vi "索引数据.vi"(6 "引用簇":T1, 7 "簇输入":cluster{"数据":T3[], "显示数据":i32[]}, 8 "错误输入（无错误）":errorcluster) -> (0 "错误输出":errorcluster, 1 "突变电压":i32, 2 "测试类型":T2, 4 "数据":dbl[][](array[numeric]), 5 "簇输出":cluster{"数据":T3[], "显示数据":i32[]})   [LabVIEW 2021]
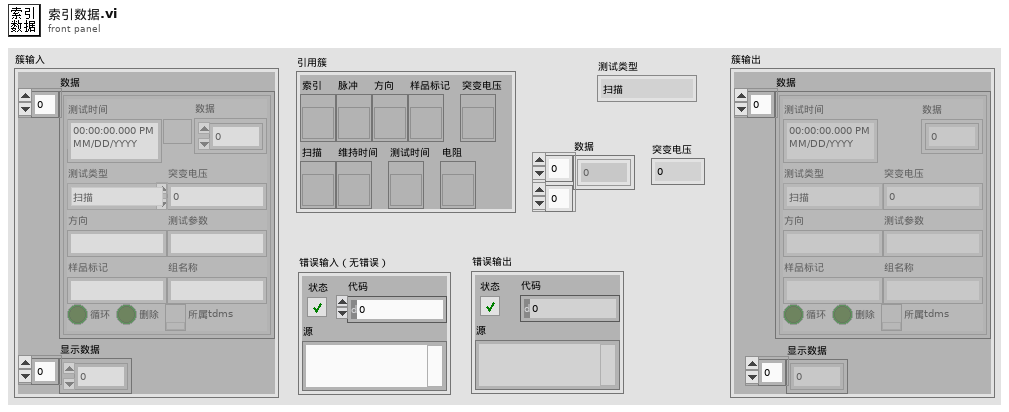
[diagram p1: front panel]
types:
  T1 = cluster{"索引":refnum<vi>, "扫描":refnum<vi>, "脉冲":refnum<vi>, "维持时间":refnum<vi>, "方向":refnum<vi>, "测试时间":refnum<vi>, "样品标记":refnum<vi>, "电阻":refnum<vi>, "突变电压":refnum<vi>}
  T2 = typedef "测试类型.ctl" = enum16{"扫描", "脉冲", "维持时间"}
  T3 = typedef "测试数据类型.ctl" = cluster{"测试时间":timestamp, "测试类型":T2, "方向":string, "样品标记":string, "测试参数":string, "循环":bool, "删除":bool, "组名称":string, "所属tdms":refnum<k34>, "突变电压":i32, "数据":dbl[][]}
  T4 = typedef "扫描参数.ctl" = cluster{"测试参数":cluster{"正向电压(V)":dbl, "正向极限电流(mA)":dbl, "反向电压(V)":dbl, "反向极限电流(mA)":dbl}, "时序参数":cluster{"正改变量(V)":dbl, "反改变量(V)":dbl, "维持时间(ms)":dbl, "nplc":dbl, "时序优先":bool}}
  T5 = typedef "脉冲参数.ctl" = cluster{"测试参数":cluster{"正向电压(V)":dbl, "正向极限电流(mA)":dbl, "反向电压(V)":dbl, "反向极限电流(mA)":dbl, "读取电压(V)":dbl}, "时序参数":cluster{"脉冲宽度(ms)":dbl, "脉冲间隔(ms)":dbl, "读取次数":u32}}
  T6 = typedef "维持时间.ctl" = cluster{"测试参数":cluster{"读取电压(V)":dbl, "极限电流(mA)":dbl}, "时序参数":cluster{"测试时间(s)":dbl, "读取间隔(ms)":dbl, "nplc":dbl, "时序优先":bool}}
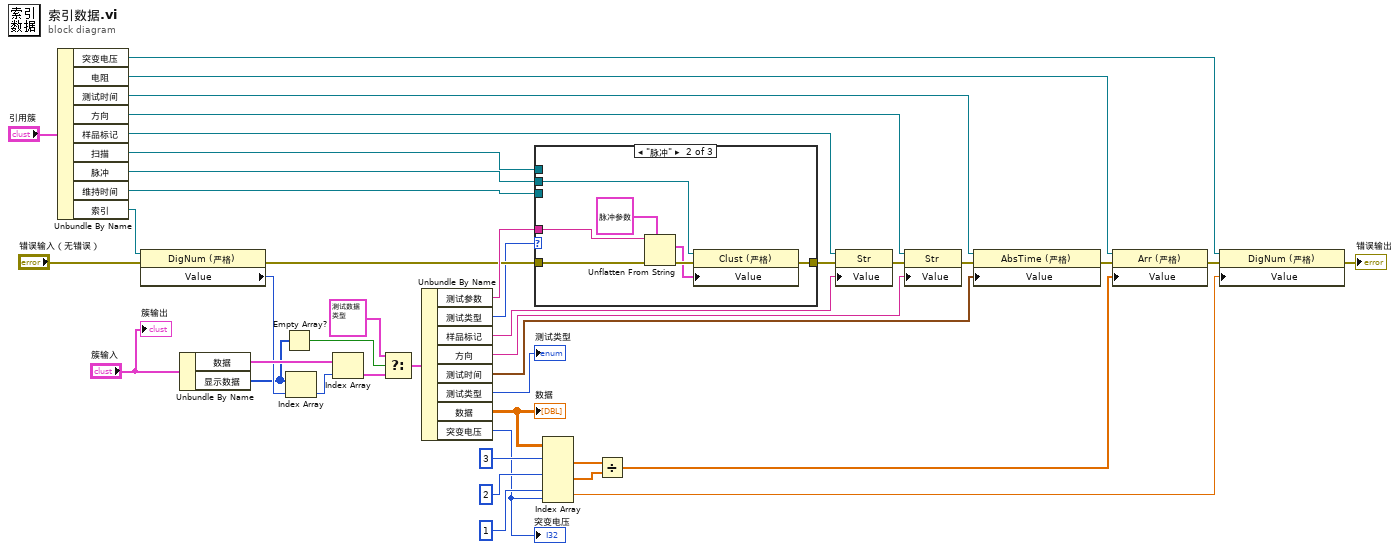
[diagram p0: block diagram]
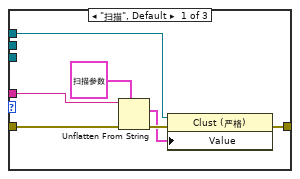
[diagram p2: hidden frame]
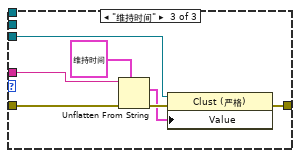
[diagram p3: hidden frame]
diagram:
  n1 = Unbundle By Name("引用簇") -> ("突变电压"=w12:refnum<vi>, "电阻"=w15:refnum<vi>, "测试时间"=w18:refnum<vi>, "方向"=w20:refnum<vi>, "样品标记"=w23:refnum<vi>, "扫描"=w29:refnum<vi>, "脉冲"=w28:refnum<vi>, "维持时间"=w27:refnum<vi>, "索引"=w24:refnum<vi>)
  n2 = property class="DigNum (严格)"(reference=w24, error in="错误输入（无错误）") -> (error out=w30:errorcluster, "Value"=w31:i32)  [unwired: 1 out]
  n3 = Unbundle By Name("簇输入") -> ("数据"=w41:T3[], "显示数据"=w4:i32[])
  n4 = Empty Array?(array=w4) -> (empty?=w3:bool)
  n5 = Index Array(array=w4, index=w31) -> (element=w42:i32)
  n6 = Index Array(array=w41, index=w42) -> (element=w5:T3)
  n7 = Select(t=T3 {"测试时间"=timestamp(0 s since 1904-01-01), "测试类型"=enum."脉冲", "方向"="", "样品标记"="", "测试参数"="\u0000\u0000\u0000\u0000\u0000\u0000\u0000\u0000\u0000\u0000\u0000\u0000\u0000\u0000\u0000\u0000\u0000\u0000\u0000\u0000\u0000\u0000\u0000\u0000\u0000\u0000\u0000\u0000\u0000\u0000\u0000\u0000\u0000\u0000\u0000\u0000\u0000\u0000\u0000\u0000\u0000\u0000\u0000\u0000\u0000\u0000\u0000\u0000\u0000\u0000\u0000\u0000", "循环"=FALSE, "删除"=FALSE, "组名称"="", "所属tdms"=refnum, "突变电压"=0, "数据"=[]}, s=w3, f=w5) -> (s? t:f=w6:T3)
  n8 = Unbundle By Name(w6) -> ("测试参数"=w38:string, "测试类型"=w8:T2, "样品标记"=w22:string, "方向"=w21:string, "测试时间"=w16:timestamp, "测试类型"=→"测试类型":T2, "数据"=w7:dbl[][], "突变电压"=w33:i32)
  "突变电压" <- w33
  "数据" <- w7
  n9 = case shown="\"脉冲\"" w8 {
    tunnel: w30 -> [w48 w55 w62]
    tunnel: [w45 w52 w59] -> w26
    tunnel: w38 -> [w46 w53 w60]
    tunnel: w29 -> [w44 _ _]
    tunnel: w28 -> [_ w51 _]
    tunnel: w27 -> [_ _ w58]
    frame "扫描", Default {
      n10 = Unflatten From String(type=T4 {"测试参数"={"正向电压(V)"=0.0, "正向极限电流(mA)"=0.0, "反向电压(V)"=0.0, "反向极限电流(mA)"=0.0}, "时序参数"={"正改变量(V)"=0.0, "反改变量(V)"=0.0, "维持时间(ms)"=0.0, "nplc"=0.0, "时序优先"=FALSE}} ("扫描"), binary string=w46, error in (no error)=w48) -> (value=w43:T4, error out=w47:errorcluster)  [unwired: 2 in, 1 out]
      n11 = property class="Clust (严格)"(reference=w44, error in=w47, "Value"=w43) -> (error out=w45:errorcluster)  [unwired: 1 out]
    }
    frame "脉冲" {
      n12 = Unflatten From String(type=T5 {"测试参数"={"正向电压(V)"=0.0, "正向极限电流(mA)"=0.0, "反向电压(V)"=0.0, "反向极限电流(mA)"=0.0, "读取电压(V)"=0.0}, "时序参数"={"脉冲宽度(ms)"=0.0, "脉冲间隔(ms)"=0.0, "读取次数"=0}} ("脉冲"), binary string=w53, error in (no error)=w55) -> (value=w50:T5, error out=w54:errorcluster)  [unwired: 2 in, 1 out]
      n13 = property class="Clust (严格)"(reference=w51, error in=w54, "Value"=w50) -> (error out=w52:errorcluster)  [unwired: 1 out]
    }
    frame "维持时间" {
      n14 = Unflatten From String(type=T6 {"测试参数"={"读取电压(V)"=0.0, "极限电流(mA)"=0.0}, "时序参数"={"测试时间(s)"=0.0, "读取间隔(ms)"=0.0, "nplc"=0.001, "时序优先"=FALSE}} ("数据"), binary string=w60, error in (no error)=w62) -> (value=w57:T6, error out=w61:errorcluster)  [unwired: 2 in, 1 out]
      n15 = property class="Clust (严格)"(reference=w58, error in=w61, "Value"=w57) -> (error out=w59:errorcluster)  [unwired: 1 out]
    }
  }
  n16 = Index Array(array=w7, index (row) #1=3 ("索引 (行)"), index (row) #2=2 ("禁用的索引 (列)"), index (row) #3=1 ("索引 (行)"), index (col) #3=w33) -> (element #1=w35:dbl[], element #2=w34:dbl[], element #3=w11:dbl)  [unwired: 2 in]
  n17 = Divide(x=w35, y=w34) -> (x/y=w14:dbl[])
  n18 = property class="Str"(reference=w23, error in=w26, "Value"=w22) -> (error out=w19:errorcluster)  [unwired: 1 out]
  n19 = property class="Str"(reference=w20, error in=w19, "Value"=w21) -> (error out=w17:errorcluster)  [unwired: 1 out]
  n20 = property class="AbsTime (严格)"(reference=w18, error in=w17, "Value"=w16) -> (error out=w13:errorcluster)  [unwired: 1 out]
  n21 = property class="Arr (严格)"(reference=w15, error in=w13, "Value"=w14) -> (error out=w10:errorcluster)  [unwired: 1 out]
  n22 = property class="DigNum (严格)"(reference=w12, error in=w10, "Value"=w11) -> (error out=→"错误输出":errorcluster)  [unwired: 1 out]
  "簇输出" <- "簇输入"
